vi "Start Test - Establish Connection.vi"(0 "Ports to Check":T4, 1 "Connection Established?":bool, 2 "Stop":bool, 3 "error in (no error)":errorcluster) -> (7 "Results":T1, 8 "Test Finished?":bool, 10 "error out":errorcluster)   [LabVIEW 2019]
doc: "Tests ports in direction of cliend to server"
uses:
  controls/Ports to Check.ctl
  controls/Results.ctl
  controls/Log Data Cluster.ctl
  controls/Communication Types.ctl
panel:
  in  "Message to Send":string="CONNECTION ESTABLISHED: You are currently accessing TCP Named Service - Server.vi from client %s on port %d."
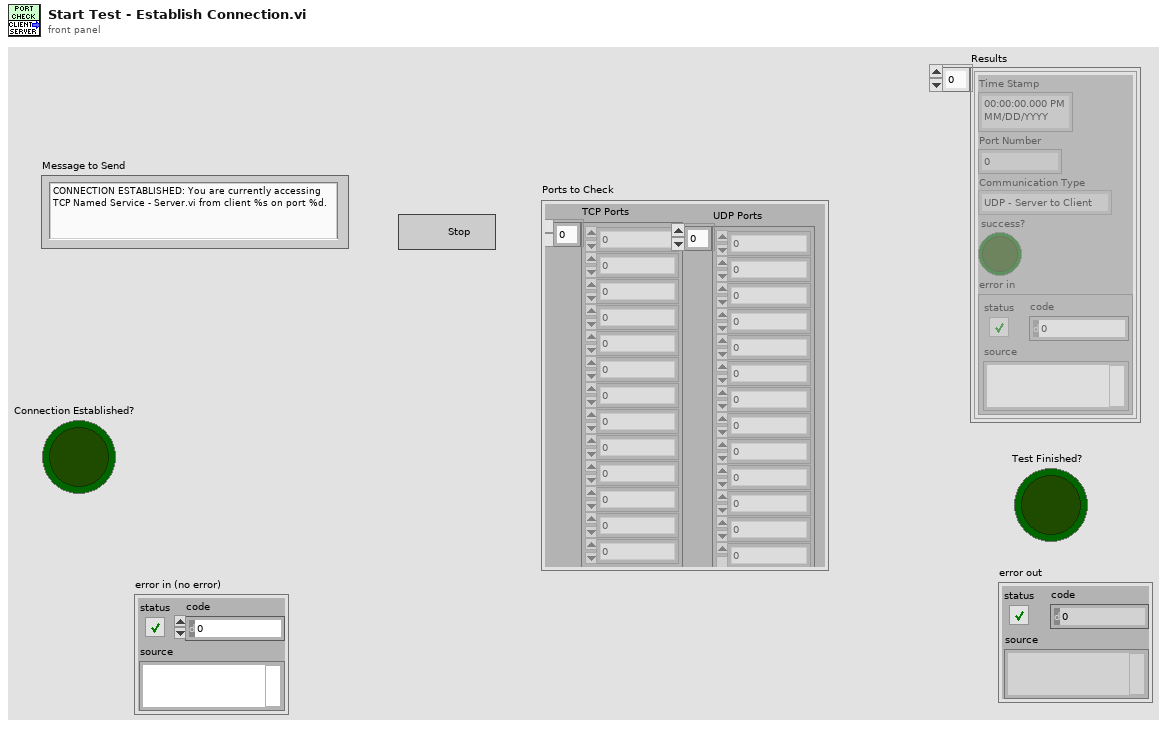
[diagram p1: front panel]
types:
  T1 = typedef "Results.ctl" = T2[]
  T2 = typedef "log data cluster.ctl" = cluster{"Time Stamp":timestamp, "Port Number":u16, "Communication Type":T3, "success?":bool, "error in":errorcluster}
  T3 = typedef "Communication Types.ctl" = enum16{"UDP - Server to Client", "UDP - Client to Server", "TCP - Server to Client", "TCP - Client to Server"}
  T4 = typedef "Ports to Check.ctl" = cluster{"TCP Ports":u32[], "UDP Ports":u32[]}
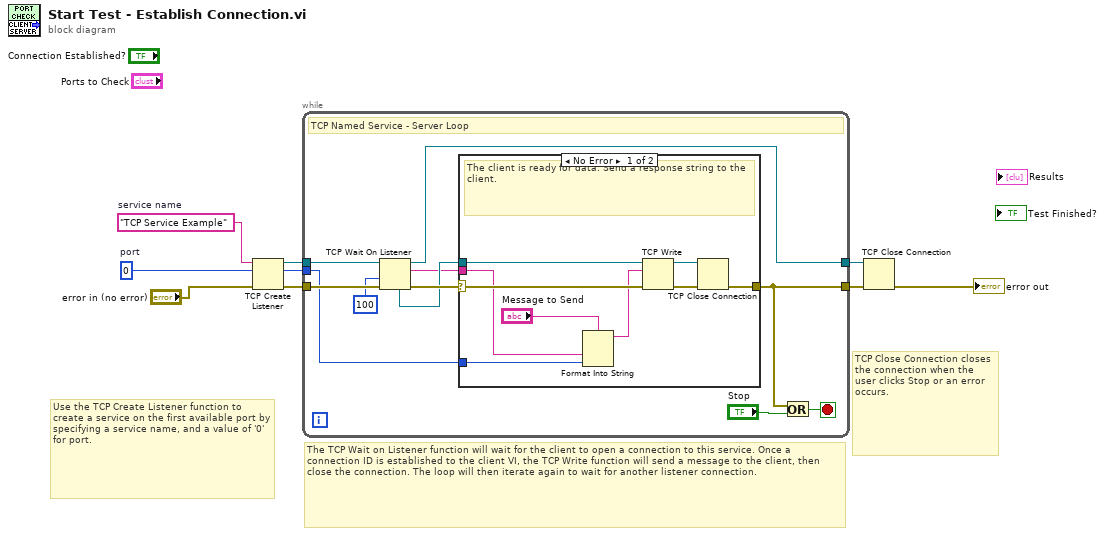
[diagram p0: block diagram]
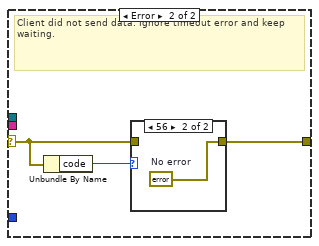
[diagram p2: hidden frame]
diagram:
  w4 = u16 0  # port
  w3 = "TCP Service Example"  # service name
  # "TCP Close Connection closes the connection when the user clicks Stop or an error occurs."
  # "The TCP Wait on Listener function will wait for the client to open a connection to this service. Once a connection ID is established to the client VI, the TCP Write function will send a message to the client, then close the connection. The loop will then iterate again to wait for another listener connection."
  # "Use the TCP Create Listener function to create a service on the first available port by specifying a service name, and a value of '0' for port."
  n1 = TCP Create Listener(8:"error in (no error)", 10:w4, 11:w3) -> (0:w8:errorcluster, 2:w5:u16, 3:w9:refnum<k5>)  [unwired: 2 in]
  n2 = while {
    tunnel: [w13] -> w6
    tunnel: w9 -> [w20]
    tunnel: w8 -> [w18]
    tunnel: [w10] -> w7
    tunnel: w5 -> [w16]
    stop <- w15 stop-if-true
    # "TCP Named Service - Server Loop"
    n3 = TCP Wait On Listener(8:w18, 9:100 ("timeout ms (25000)"), 11:w20) -> (0:w19:errorcluster, 2:w11:string, 3:w10:refnum<k5>, 4:w17:refnum<k5>)  [unwired: 1 in, 1 out]
    n4 = case shown="No Error" w19 {
      selector: w19 -> [w29 w32]
      tunnel: [w22 w30] -> w13
      tunnel: w17 -> [w23 _]
      tunnel: w16 -> [w27 _]
      tunnel: w11 -> [w25 _]
      frame No Error {
        # "The client is ready for data. Send a response string to the client."
        n5 = Format Into String(format string="Message to Send", w25, w27) -> (resulting string=w24:string)  [unwired: 2 in, 1 out]
        n6 = TCP Write(connection ID=w23, data in=w24, error in (no error)=w29) -> (connection ID out=w21:refnum<k5>, error out=w28:errorcluster)  [unwired: 1 in, 1 out]
        n7 = TCP Close Connection(connection ID=w21, error in (no error)=w28) -> (error out=w22:errorcluster)  [unwired: 1 in, 1 out]
      }
      frame Error {
        # "Client did not send data. Ignore timeout error and keep waiting."
        n8 = Unbundle By Name(w32) -> ("code"=w31:i32)
        n9 = case shown="56" w31 {
          tunnel: w32 -> [w33 _]
          tunnel: [w33 w34] -> w30
          frame Default {
          }
          frame 56 {
            w34 = errorcluster {"status"=FALSE, "code"=0, "source"=""}  # No error
          }
        }
      }
    }
    n10 = Or(x=w13, y="Stop") -> (x .or. y?=w15:bool)
  }
  n11 = TCP Close Connection(connection ID=w7, error in (no error)=w6) -> (error out=→"error out":errorcluster)  [unwired: 1 in, 1 out]
